vi "Drivetrain Trapezoidal Loop.vi"(9 "Axes":T1) -> (1 "Shift?":bool, 2 "Y Power":dbl)   [LabVIEW 2017]
uses:
  Robot Global Data.vi
  Common Code/Trapezoidal States.ctl
  <vilib>/addons/control/pid/NI_PID_pid.lvlib
  <vilib>/addons/control/pid/pid.llb/PID (DBL).vi
  <vilib>/express/express arith-compare/Formula/XNode/ExpressFormulaBlockNode.xnode
  Common Code/Gamepads/Axes Cluster.ctl
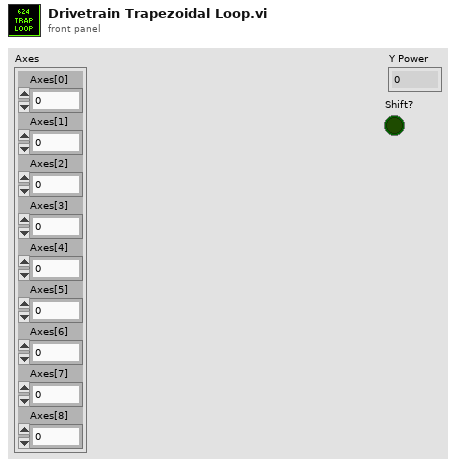
[diagram p1: front panel]
types:
  T1 = typedef "Axes Cluster.ctl" = cluster{"Axes[0]":dbl, "Axes[1]":dbl, "Axes[2]":dbl, "Axes[3]":dbl, "Axes[4]":dbl, "Axes[5]":dbl, "Axes[6]":dbl, "Axes[7]":dbl, "Axes[8]":dbl}
  T2 = typedef "Trapezoidal States.ctl" = enum16{"Feed Forward", "Feed Backwards", "Cruise", "Shift Feed Forward", "Shift Feed Backwards", "Shift Cruise", "Idle"}
  T3 = typedef "Dashboard Control Data.ctl" = cluster{"Drivetrain Settings Cluster":T4, "Intake Presets":T9, "Elevator Settings Cluster":T10, "Drivetrain Encoder Values":T12, "Auton Chooser":T13, "Auton Presets":cluster{"Start Position":dbl}, "Elevator Encoder Values":T14, "Pressure M":dbl, "Pressure B":dbl, "Zero All?":bool, "Enable Vision":bool}
  T4 = typedef "Drivetrain Settings Cluster.ctl" = cluster{"Gyro Steer PID Gains":T5, "Distance Drive PID Gains":T5, "Drive Tolerance":dbl, "Gyro Tolerance":dbl, "Gyro Output":dbl, "Distance Output":dbl, "Y Power Multiplier":dbl, "Turn Power Multiplier":dbl, "Creep Rate":dbl, "Encoder Reset":bool, "DT Mode Modifier":enum16{"None, Default", "Cube", "Square"}, "Left Encoder Tick Constant":dbl, "Right Encoder Tick Constant":dbl, "Shift Speed":dbl, "Zero Gyro":bool, "Y min":dbl, "Y max":dbl, "X min":dbl, "X max":dbl, "Finish Velocity":dbl, "Anti-Tip Settings":T6, "Trapezoidal Settings":T7, "Turning, Don't Shift":dbl}
  T5 = typedef "PID Gains Cluster.ctl" = cluster{"Proportional Gain":dbl, "Integral Time":dbl, "Derivative Time":dbl}
  T6 = typedef "Anti-Tip Settings.ctl" = cluster{"Pitch Tip Constant":dbl, "Wheel Diameter":dbl, "Gearbox Reduction":dbl, "Motor Count":dbl, "Mass of Robot":dbl, "Almost Tip Constant":dbl, "Dist to CG":dbl}
  T7 = typedef "Trapezoidal Settings.ctl" = cluster{"1st Gear Reduction":dbl, "2nd Gear Reduction":dbl, "Maximum RPM":dbl, "1st Gear PVA Gains":T8, "2nd Gear PVA Gains":T8, "Wheel Radius":dbl, "Mass of the Wheel":dbl, "Number of Motors":dbl, "Velocity Tolerance":dbl, "Cruise Time (ms)":dbl, "Efficiency":dbl}
  T8 = typedef "PVA Gains.ctl" = cluster{"Positional Gain":dbl, "Velocity Gain":dbl, "Acceleration Gain":dbl}
  T9 = typedef "Intake Presets.ctl" = cluster{"Idle Angle":dbl, "Mid Angle":dbl, "Low Angle":dbl, "Outtake Power":dbl, "Intake Power":dbl, "Unstuck":dbl, "Angle Tolerance":dbl, "Max Angle":dbl, "Max Current":dbl, "Current Trip Time":dbl, "Reset Encoder?":bool, "Encoder Scale":dbl, "PID gains":cluster{"proportional gain (Kc)":dbl, "integral time (Ti, min)":dbl, "derivative time (Td, min)":dbl}, "output range":cluster{"output high":dbl, "output low":dbl}, "IR Constant Pull Rate":dbl, "Shoot Angle":dbl, "Shoot High":dbl, "Manual Limit":dbl}
  T10 = typedef "Elevator Settings Cluster.ctl" = cluster{"Ground Height":dbl, "Switch Height":dbl, "Scale High Height ":dbl, "Scale Low Height":dbl, "Elevator PID Gains":T11, "Elevator Tolerance":dbl, "Reset Encoders":bool, "Encoder Scale":dbl, "Max Height":dbl, "Mid Height":dbl, "output range":cluster{"output high":dbl, "output low":dbl}, "Upper Slow Down Tolerance":dbl, "Tick Constant":dbl, "Tip Constant":dbl, "Slow Down Multiplier":dbl, "Almost Tip Constant":dbl, "Bottom Trip Offset":dbl, "Lower Slow Down Tolerance":dbl, "Cruise Velocity":dbl, "Max Acceleration":dbl, "Feed Forward":dbl}
  T11 = typedef "PID Gains.ctl" = cluster{"proportional gain (Kc)":dbl, "integral time (Ti, min)":dbl, "derivative time (Td, min)":dbl}
  T12 = typedef "DT Encoder Values.ctl" = cluster{"Left Encoder":cluster{"Distance":dbl, "Speed":dbl, "Tick":dbl}, "Right Encoder":cluster{"Distance":dbl, "Speed":dbl, "Tick":dbl}}
  T13 = typedef "Auton Chooser.ctl" = cluster{"Left":bool, "Center":bool, "Right":bool, "Scale":bool, "Both":bool, "Switch":bool, "Test":bool, "No Script":bool, "Drive PID":bool, "Elevator PID":bool, "Gyro PID":bool, "Drive Forward":bool, "cross front":bool, "Near":bool, "Far":bool, "1 Plus 1":bool, "2 Scale":bool, "2 Switch":bool, "cross behind":bool, "Pick up 2nd cube":bool, "No cross if cross":bool}
  T14 = typedef "Elevator Encoder Values.ctl" = cluster{"Encoder Values":cluster{"Distance":dbl, "Speed":dbl, "Tick":dbl}}
  T15 = typedef "Dashboard Status Data.ctl" = cluster{"Elevator Status Cluster":T16, "Drivetrain Status Cluster":T19, "Intake Status Cluster":T21, "Climb Status Cluster":T24, "Intake PDP Info":T25, "Auton Command Cluster":T26, "Pressure ":dbl, "Auton Field Index":i32, "Auton File Index":i32, "Auton Side Index":i32, "Auton Side":string, "Field Config":string, "Robot Info":T27, "IMU Pitch Zero":dbl, "IMU Roll Zero":dbl, "IMU Yaw Zero":dbl, "Auton Queue Index":i32}
  T16 = typedef "Elevator Status Cluster.ctl" = cluster{"Finished":bool, "Elevator Power":dbl, "Elevator State":T17, "Elevator Mode":T18, "Elevator Height":dbl, "At Bottom?":bool, "At Top?":bool, "Scale high?":bool, "PID Output":dbl, "2nd Gear":bool}
  T17 = typedef "Elevator State.ctl" = enum16{"Idle", "Ground", "Mid", "Scale", "Switch"}
  T18 = typedef "Elevator Mode.ctl" = enum16{"Motion Profile", "Semi Auto", "Manual", "Auto"}
  T19 = typedef "Drivetrain Status Cluster.ctl" = cluster{"Throttle (Y)":dbl, "Steer (X)":dbl, "Drivetrain Mode":T20, "Brake?":bool, "Distance Drive Complete?":bool, "PID Drive Complete?":bool, "Creep Mode?":bool, "Gyro Steer Complete?":bool, "Gyro":dbl, "Heading Target":dbl, "Distance Target":dbl, "2nd Gear":bool, "Drivetrain Encoder Values":T12, "Left Motor Power":dbl, "Right Motor Power":dbl}
  T20 = typedef "Drivetrain Mode.ctl" = enum16{"Manual w/ Autoshift", "Trapezoidal Motion", "Manual", "Gyro Steer", "PID Drive", "Distance Drive", "Autonomous"}
  T21 = typedef "Intake Status Cluster.ctl" = cluster{"Intake Mode":T22, "Intake States":T23, "Intake Current Angle":dbl, "Cube In Posession?":bool, "Intake Wrist Up?":bool, "Right Roller Power":dbl, "Angle Power":dbl, "Left Roller Power":dbl}
  T22 = typedef "Intake Mode.ctl" = enum16{"Auto", "Semi Auto", "Manual"}
  T23 = typedef "Intake States.ctl" = enum16{"Zero", "Override Angle", "Idle", "Drop Mid", "Drop Low", "Outtake", "Intake"}
  T24 = typedef "Climb Status Cluster.ctl" = cluster{"Climb":bool, "Time Remaining":dbl, "Button Pressed":bool}
  T25 = typedef "Intake PDP Info.ctl" = cluster{"Voltage Percent Output":dbl, "Output Voltage":dbl, "Bus Voltage":dbl, "Device ID":dbl, "Output Current":dbl, "Sensor Velocity":dbl, "Sensor Position":dbl, "Pulse Width Position":dbl, "Pulse Width Velocity":dbl, "Temperature":dbl, "Inverted?":bool}
  T26 = typedef "Auton Command Cluster.ctl" = cluster{"commandID":dbl, "headingTarget":dbl, "async":dbl, "elevatorCommand":dbl, "intakeMode":dbl, "maxTime":dbl, "ySpeed":dbl, "zeroGyro":dbl, "intakeCommand":dbl, "distanceTarget":dbl, "xSpeed":dbl, "elevatorMode":dbl, "scaleHigh":dbl, "rollerSpeed":dbl, "intakeAngle":dbl, "manualOpen":dbl, "secondGear":dbl, "elevatorPower":dbl, "waitFor":dbl, "overrideAngle":dbl}
  T27 = typedef "Robot Info.ctl" = cluster{"FMS":bool, "Switch and Scale Sides":string, "Event Name":string, "Alliance":T28, "Position":T29, "Match Number":u16, "Robot Mode":T30, "Match Time(s)":sgl}
  T28 = typedef "WPI_DriverStationAllianceInfo.ctl" = enum16{"Red", "Blue", "Invalid"}
  T29 = typedef "WPI_DriverStationPositionInfo.ctl" = enum16{"1", "2", "3"}
  T30 = typedef "WPI_DriverStationRobotMode2.ctl" = enum16{"Autonomous Disabled", "Autonomous Enabled", "Teleop Disabled", "Teleop Enabled", "Disconnected", "Finish", "Test Disabled", "Test Enabled", "Emergency Stopped"}
  T31 = typedef "Drivetrain Command Cluster.ctl" = cluster{"Y Power":dbl, "Turn Power":dbl, "Drivetrain Mode":T20, "2nd Gear":bool, "Y Min Output":dbl, "Y Max Output":dbl, "X Min Output":dbl, "X Max Output":dbl, "Heading Target":dbl, "Distance Target":dbl, "Brake?":bool, "Zero Gyro":bool, "Trapezoidal States":T2}
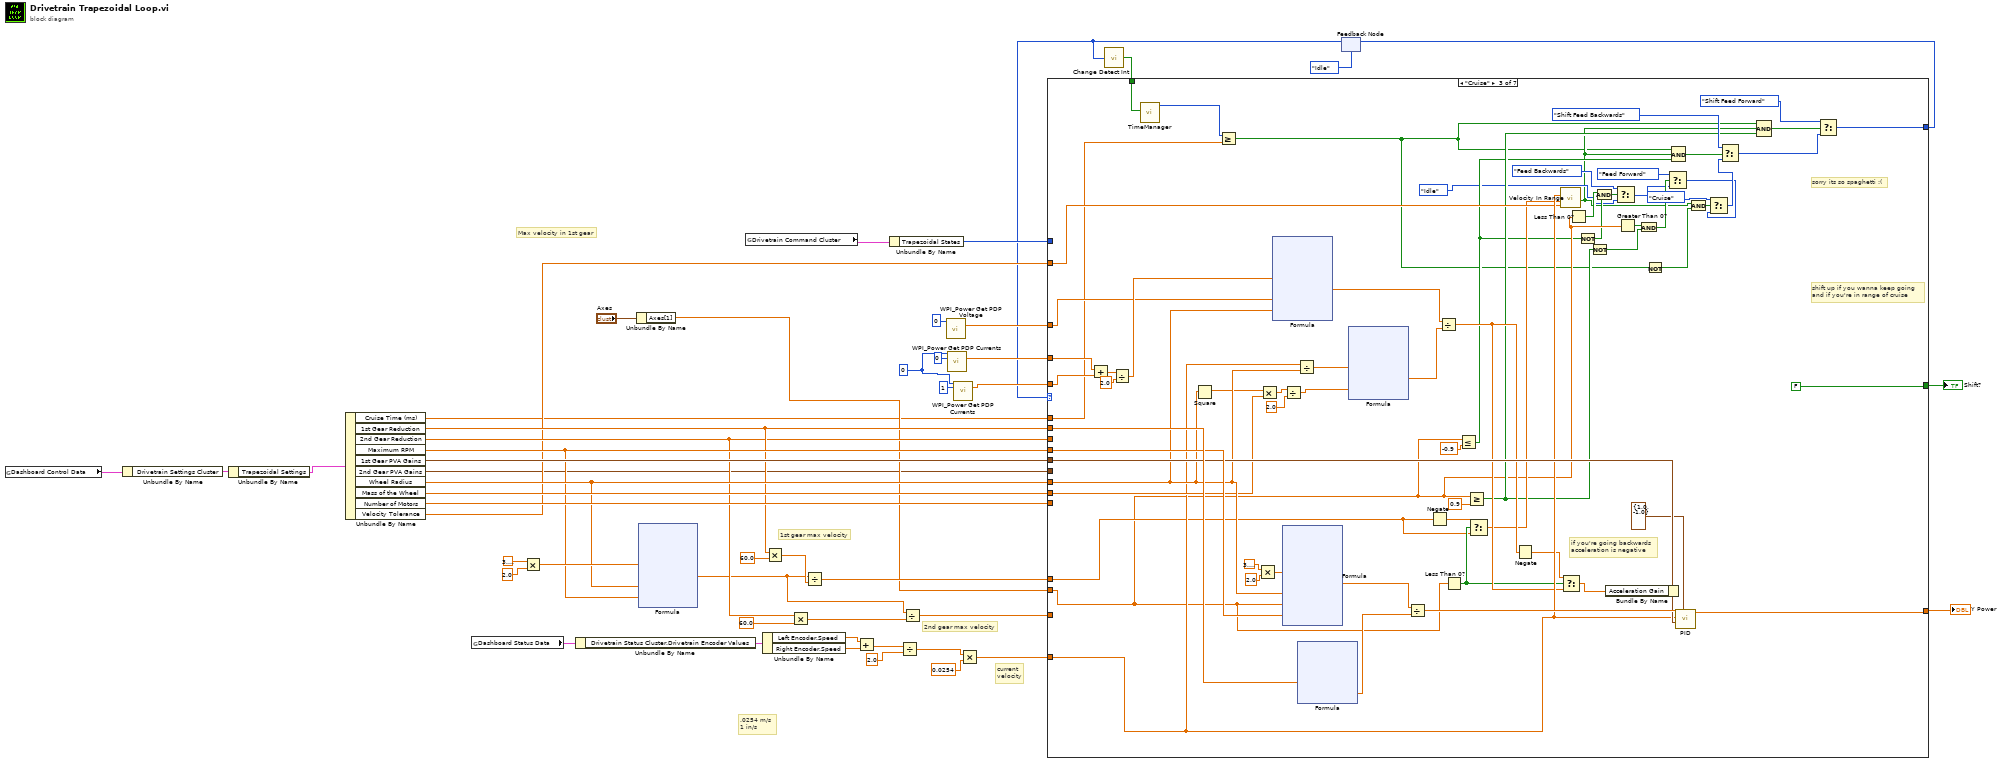
[diagram p0: block diagram]
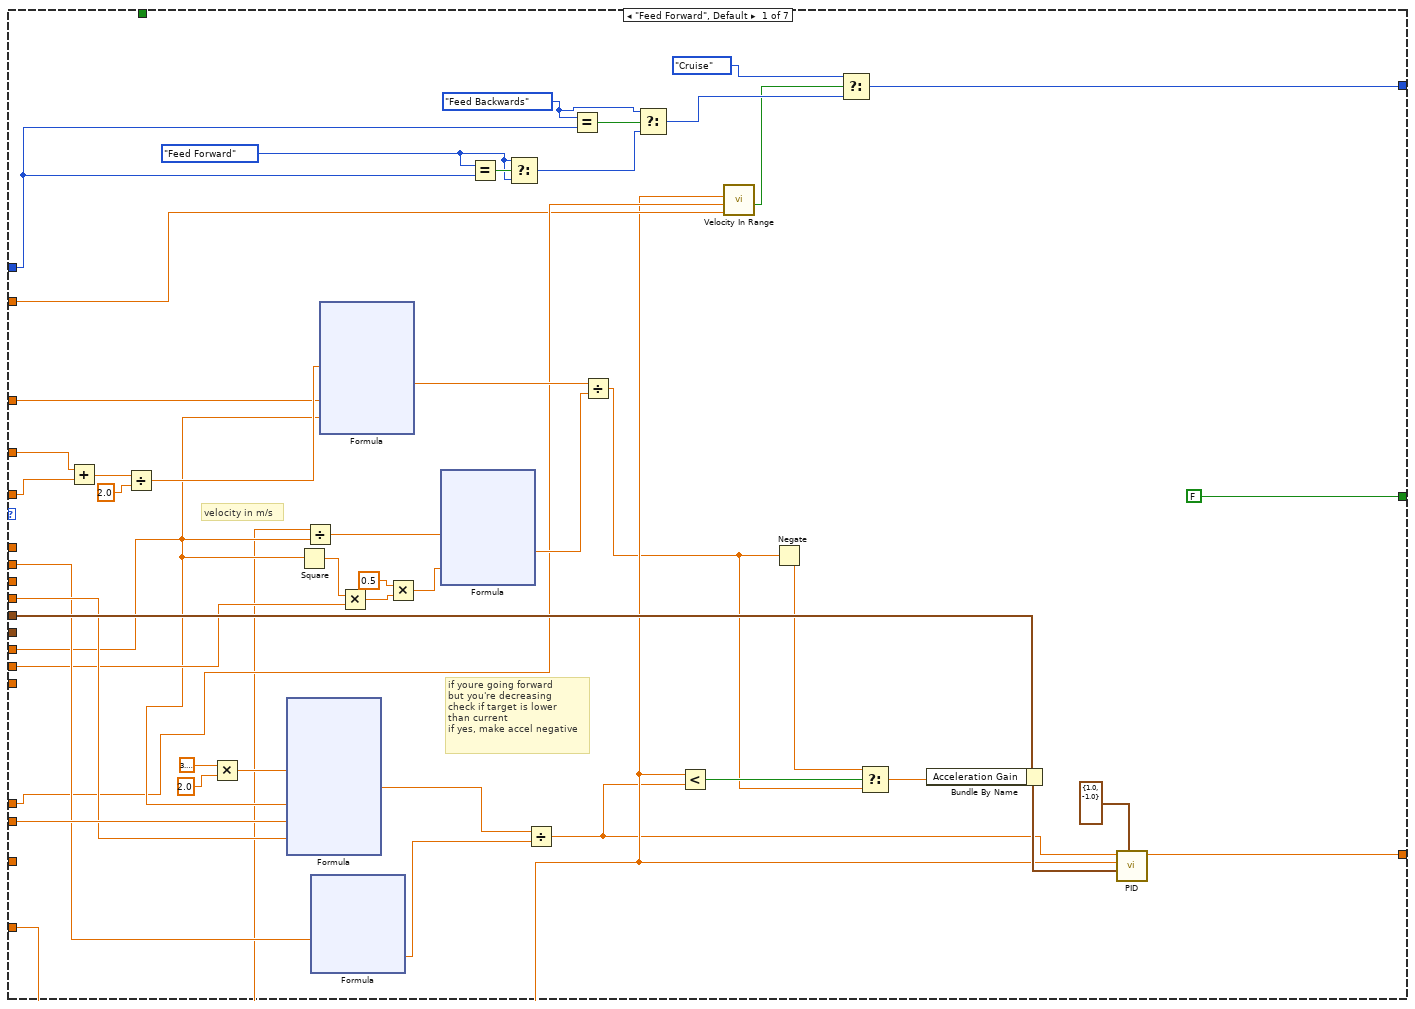
[diagram p2: hidden frame]
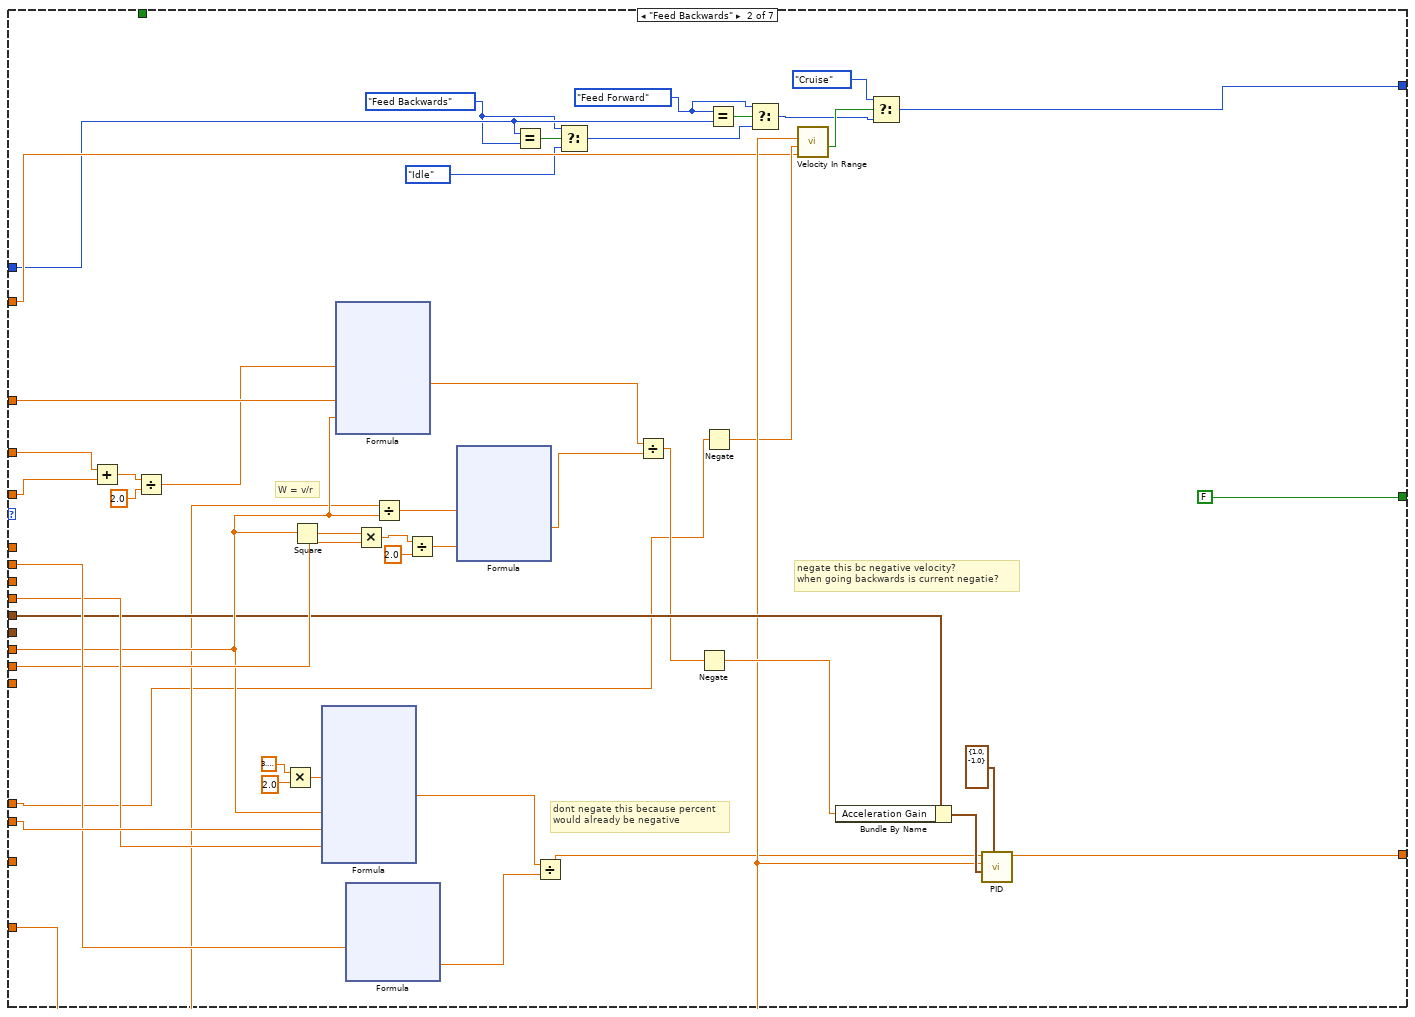
[diagram p3: hidden frame]
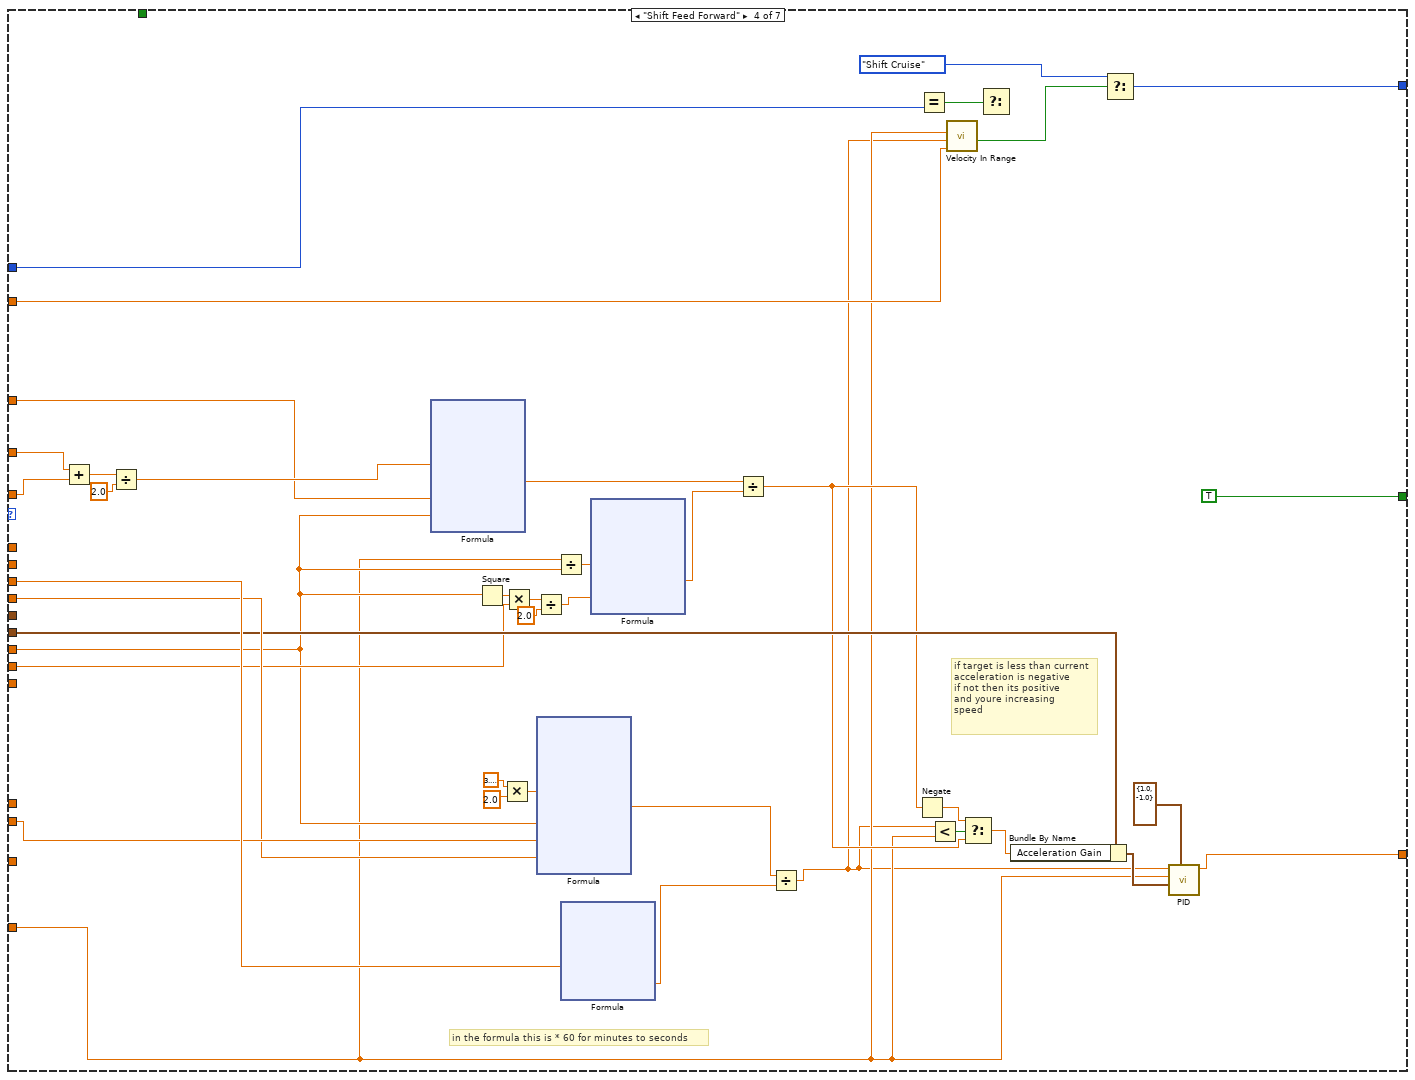
[diagram p4: hidden frame]
diagram:
  w27 = 0
  # "current\nvelocity"
  # "2nd gear max velocity"
  # "1st gear max velocity"
  # "Max velocity in 1st gear"
  # ".0254 m/s \n1 in/s"
  n1 = global read "Robot Global Data.vi" "Dashboard Control Data"() -> (w49:T3)
  n2 = Unbundle By Name(w49) -> ("Drivetrain Settings Cluster"=w48:T4)
  n3 = Unbundle By Name(w48) -> ("Trapezoidal Settings"=w47:T7)
  n4 = Unbundle By Name(w47) -> ("Cruise Time (ms)"=w2:dbl, "1st Gear Reduction"=w19:dbl, "2nd Gear Reduction"=w15:dbl, "Maximum RPM"=w20:dbl, "1st Gear PVA Gains"=w44:T8, "2nd Gear PVA Gains"=w1:T8, "Wheel Radius"=w21:dbl, "Mass of the Wheel"=w43:dbl, "Number of Motors"=w34:dbl, "Velocity Tolerance"=w6:dbl)
  n5 = global read "Robot Global Data.vi" "Dashboard Status Data"() -> (w42:T15)
  n6 = Multiply(x=3.141592653589793, y=2.0) -> (x*y=w23:dbl)
  n7 = Unbundle By Name(w42) -> ("Drivetrain Status Cluster.Drivetrain Encoder Values"=w41:T12)
  n8 = Unbundle By Name("Axes") -> ("Axes[1]"=w8:dbl)
  n9 = xnode "Formula"("2PI"=w23, "Wheel Radius"=w21, "Max RPM"=w20) -> ("Result"=w13:dbl)  [unwired: 1 in, 1 out]
  n10 = global read "Robot Global Data.vi" "Drivetrain Command Cluster"() -> (w46:T31)
  n11 = Unbundle By Name(w41) -> ("Left Encoder.Speed"=w40:dbl, "Right Encoder.Speed"=w39:dbl)
  n12 = Multiply(x=w19, y=60.0) -> (x*y=w17:dbl)
  n13 = Multiply(x=w15, y=60.0) -> (x*y=w12:dbl)
  n14 = Divide(x=w13, y=w17) -> (x/y=w16:dbl)
  n15 = Add(x=w40, y=w39) -> (x+y=w38:dbl)
  n16 = Unbundle By Name(w46) -> ("Trapezoidal States"=w25:T2)
  n17 = Divide(x=w38, y=2.0) -> (x/y=w36:dbl)
  n18 = Divide(x=w13, y=w12) -> (x/y=w11:dbl)
  n19 = call <vilib>:"WPI_Power Get PDP Voltage.vi"("Power Distribution Panel (0)"=u8 0) -> ("voltage (V)"=w31:dbl)  [unwired: 13 in, 1 out]
  n20 = call <vilib>:"WPI_Power Get PDP Currents.vi"("Power Distribution Panel (0)"=w27, "PDP Channel"=0) -> ("current (A)"=w32:dbl)  [unwired: 11 in, 2 out]
  n21 = call <vilib>:"WPI_Power Get PDP Currents.vi"("Power Distribution Panel (0)"=w27, "PDP Channel"=1) -> ("current (A)"=w26:dbl)  [unwired: 11 in, 2 out]
  n22 = Multiply(x=w36, y=0.0254) -> (x*y=w33:dbl)
  n23 = feedback #1(Trapezoidal_States."Idle" ("Trapezoidal States")) -> (w4:T2)
  n24 = call "Change Detect Int.vi"("In"=w4) -> ("Changed?"=w3:bool)
  n25 = case shown="\"Cruise\"" w4 {
    tunnel: w44 -> [w94 w162 w287 _ _ _ _]
    tunnel: w21 -> [w74 w164 w279 w356 _ _ _]
    tunnel: w43 -> [w77 w167 w277 w358 _ _ _]
    tunnel: w20 -> [w89 w179 w295 w375 _ _ _]
    tunnel: w15 -> [_ _ _ w380 _ _ _]
    tunnel: w19 -> [w87 w180 w296 _ _ _ _]
    tunnel: w8 -> [w90 w181 w244 w376 _ _ _]
    tunnel: w34 -> [_ _ _ _ _ _ _]
    tunnel: w33 -> [w55 w155 w271 w345 _ _ _]
    tunnel: w32 -> [w84 w175 w286 w368 _ _ _]
    tunnel: w31 -> [w79 w176 w281 w357 _ _ _]
    tunnel: w26 -> [w83 w174 w285 w367 _ _ _]
    tunnel: w25 -> [w70 w145 _ w342 _ _ _]
    tunnel: w16 -> [w59 w154 w260 _ _ _ _]
    tunnel: w11 -> [_ _ _ _ _ _ _]
    tunnel: [w65 w151 w256 w347 _ _ _] -> w10
    tunnel: [w63 w185 w297 w371 _ _ _] -> w7
    tunnel: w6 -> [w58 w152 w270 w346 _ _ _]
    tunnel: [FALSE FALSE FALSE TRUE _ _ _] -> w5
    tunnel: w3 -> [_ _ w255 _ _ _ _]
    tunnel: w2 -> [_ _ w253 _ _ _ _]
    tunnel: w1 -> [_ _ _ w369 _ _ _]
    frame "Feed Forward", Default {
      w64 = Trapezoidal_States."Feed Forward" ("Trapezoidal States")
      w68 = Trapezoidal_States."Feed Backwards" ("Trapezoidal States")
      # "if youre going forward\nbut you're decreasing\ncheck if target is lower\nthan current \nif yes, make accel negative"
      # "velocity in m/s"
      n26 = Add(x=w84, y=w83) -> (x+y=w82:dbl)
      n27 = Divide(x=w82, y=2.0) -> (x/y=w80:dbl)
      n28 = Multiply(x=3.141592653589793, y=2.0) -> (x*y=w91:dbl)
      n29 = xnode "Formula"("2PI"=w91, "Wheel Radius"=w74, "Percent Output"=w90, "Maximum RPM"=w89) -> ("Result"=w88:dbl)  [unwired: 1 in, 1 out]
      n30 = Square(x=w74) -> (x^2=w62:dbl)
      n31 = Divide(x=w55, y=w74) -> (x/y=w73:dbl)
      n32 = xnode "Formula"("Gear Reduction"=w87) -> ("Result"=w86:dbl)  [unwired: 1 in, 1 out]
      n33 = xnode "Formula"("AvgCurrent"=w80, "Voltage"=w79, "Wheel Radius"=w74) -> ("Result"=w78:dbl)  [unwired: 1 in, 1 out]
      n34 = Multiply(x=w62, y=w77) -> (x*y=w60:dbl)
      n35 = Multiply(x=0.5, y=w60) -> (x*y=w76:dbl)
      n36 = xnode "Formula"("AngularSpeed"=w73, "Inertia"=w76) -> ("Result"=w75:dbl)  [unwired: 1 in, 1 out]
      n37 = Equal?(x=w64, y=w70) -> (x = y?=w69:bool)
      n38 = Select(t=w64, s=w69, f=w64) -> (s? t:f=w66:T2)
      n39 = Divide(x=w88, y=w86) -> (x/y=w54:dbl)
      n40 = Equal?(x=w68, y=w70) -> (x = y?=w71:bool)
      n41 = Divide(x=w78, y=w75) -> (x/y=w50:dbl)
      n42 = Select(t=w68, s=w71, f=w66) -> (s? t:f=w67:T2)
      n43 = Less?(x=w55, y=w54) -> (x < y?=w53:bool)
      n44 = call "Velocity In Range.vi"("Velocity Tolerance"=w58, "Target Velocity"=w59, "Current Velocity"=w55) -> ("In Range?"=w57:bool)  [unwired: 8 in]
      n45 = Negate(x=w50) -> (-x=w52:dbl)
      n46 = Select(t=Trapezoidal_States."Cruise" ("Trapezoidal States"), s=w57, f=w67) -> (s? t:f=w65:T2)
      n47 = Select(t=w52, s=w53, f=w50) -> (s? t:f=w51:dbl)
      n48 = Bundle By Name(cluster=w94, "Acceleration Gain"=w51) -> (w95:T8)
      n49 = call-poly <vilib>:"PID.vi"("output range"=cluster{"output high":dbl, "output low":dbl} {"output high"=1.0, "output low"=-1.0}, "PID gains"=w95, "process variable"=w55, "setpoint"=w54) -> ("output"=w63:dbl)  [unwired: 6 in, 1 out]
    }
    frame "Feed Backwards" {
      w144 = Trapezoidal_States."Feed Backwards" ("Trapezoidal States")
      w148 = Trapezoidal_States."Feed Forward" ("Trapezoidal States")
      # "negate this bc negative velocity?\nwhen going backwards is current negatie?"
      # "dont negate this because percent\nwould already be negative"
      # "W = v/r"
      n50 = Add(x=w175, y=w174) -> (x+y=w173:dbl)
      n51 = Divide(x=w173, y=2.0) -> (x/y=w171:dbl)
      n52 = Multiply(x=3.141592653589793, y=2.0) -> (x*y=w183:dbl)
      n53 = Square(x=w164) -> (x^2=w168:dbl)
      n54 = xnode "Formula"("2PI"=w183, "Wheel Radius"=w164, "Percent Output"=w181, "Maximum RPM"=w179) -> ("Result"=w178:dbl)  [unwired: 1 in, 1 out]
      n55 = xnode "Formula"("AvgCurrent"=w171, "Voltage"=w176, "Wheel Radius"=w164) -> ("Result"=w160:dbl)  [unwired: 1 in, 1 out]
      n56 = xnode "Formula"("Gear Reduction"=w180) -> ("Result"=w177:dbl)  [unwired: 1 in, 1 out]
      n57 = Multiply(x=w168, y=w167) -> (x*y=w166:dbl)
      n58 = Divide(x=w155, y=w164) -> (x/y=w165:dbl)
      n59 = Divide(x=w166, y=2.0) -> (x/y=w170:dbl)
      n60 = xnode "Formula"("AngularSpeed"=w165, "Inertia"=w170) -> ("Result"=w159:dbl)  [unwired: 1 in, 1 out]
      n61 = Equal?(x=w145, y=w144) -> (x = y?=w146:bool)
      n62 = Divide(x=w178, y=w177) -> (x/y=w150:dbl)
      n63 = Select(t=w144, s=w146, f=Trapezoidal_States."Idle" ("Trapezoidal States")) -> (s? t:f=w143:T2)
      n64 = Divide(x=w160, y=w159) -> (x/y=w158:dbl)
      n65 = Negate(x=w158) -> (-x=w161:dbl)
      n66 = Negate(x=w154) -> (-x=w153:dbl)
      n67 = Equal?(x=w148, y=w145) -> (x = y?=w149:bool)
      n68 = Select(t=w148, s=w149, f=w143) -> (s? t:f=w147:T2)
      n69 = call "Velocity In Range.vi"("Velocity Tolerance"=w152, "Target Velocity"=w153, "Current Velocity"=w155) -> ("In Range?"=w156:bool)  [unwired: 8 in]
      n70 = Bundle By Name(cluster=w162, "Acceleration Gain"=w161) -> (w163:T8)
      n71 = Select(t=Trapezoidal_States."Cruise" ("Trapezoidal States"), s=w156, f=w147) -> (s? t:f=w151:T2)
      n72 = call-poly <vilib>:"PID.vi"("output range"=cluster{"output high":dbl, "output low":dbl} {"output high"=1.0, "output low"=-1.0}, "PID gains"=w163, "process variable"=w155, "setpoint"=w150) -> ("output"=w185:dbl)  [unwired: 6 in, 1 out]
    }
    frame "Cruise" {
      # "sorry its so spaghetti :("
      # "if you're going backwards\nacceleration is negative"
      # "shift up if you wanna keep going \nand if you're in range of cruise"
      n73 = Add(x=w286, y=w285) -> (x+y=w284:dbl)
      n74 = Divide(x=w284, y=2.0) -> (x/y=w282:dbl)
      n75 = call "TimeManager.vi"("Reset?"=w255) -> ("Time Since Reset"=w254:u32)  [unwired: 9 in, 1 out]
      n76 = Square(x=w279) -> (x^2=w278:dbl)
      n77 = Greater Or Equal?(x=w254, y=w253) -> (x >= y?=w234:bool)
      n78 = Multiply(x=3.141592653589793, y=2.0) -> (x*y=w294:dbl)
      n79 = Multiply(x=w278, y=w277) -> (x*y=w276:dbl)
      n80 = xnode "Formula"("AvgCurrent"=w282, "Voltage"=w281, "Wheel Radius"=w279) -> ("Result"=w273:dbl)  [unwired: 1 in, 1 out]
      n81 = xnode "Formula"("2PI"=w294, "Wheel Radius"=w279, "Percent Output"=w244, "Maximum RPM"=w295) -> ("Result"=w291:dbl)  [unwired: 1 in, 1 out]
      n82 = Divide(x=w276, y=2.0) -> (x/y=w274:dbl)
      n83 = Divide(x=w271, y=w279) -> (x/y=w280:dbl)
      n84 = xnode "Formula"("Gear Reduction"=w296) -> ("Result"=w290:dbl)  [unwired: 1 in, 1 out]
      n85 = xnode "Formula"("AngularSpeed"=w280, "Inertia"=w274) -> ("Result"=w272:dbl)  [unwired: 1 in, 1 out]
      n86 = Divide(x=w291, y=w290) -> (x/y=w289:dbl)
      n87 = Negate(x=w260) -> (-x=w261:dbl)
      n88 = Divide(x=w273, y=w272) -> (x/y=w266:dbl)
      n89 = Less Than 0?(x=w244) -> (x < 0?=w262:bool)
      n90 = Less Or Equal?(x=w244, y=-0.9) -> (x <= y?=w242:bool)
      n91 = Greater Or Equal?(x=w244, y=0.9) -> (x >= y?=w249:bool)
      n92 = Select(t=w261, s=w262, f=w260) -> (s? t:f=w259:dbl)
      n93 = Negate(x=w266) -> (-x=w267:dbl)
      n94 = call "Velocity In Range.vi"("Velocity Tolerance"=w270, "Target Velocity"=w259, "Current Velocity"=w271) -> ("In Range?"=w235:bool)  [unwired: 8 in]
      n95 = Select(t=w267, s=w262, f=w266) -> (s? t:f=w265:dbl)
      n96 = Less Than 0?(x=w244) -> (x < 0?=w243:bool)
      n97 = Not(x=w242) -> (.not. x?=w241:bool)
      n98 = Not(x=w249) -> (.not. x?=w248:bool)
      n99 = And(x=w243, y=w241) -> (x .and. y?=w245:bool)
      n100 = Bundle By Name(cluster=w287, "Acceleration Gain"=w265) -> (w288:T8)
      n101 = Select(t=Trapezoidal_States."Feed Backwards" ("Trapezoidal States"), s=w245, f=Trapezoidal_States."Idle" ("Trapezoidal States")) -> (s? t:f=w239:T2)
      n102 = Greater Than 0?(x=w244) -> (x > 0?=w250:bool)
      n103 = And(x=w250, y=w248) -> (x .and. y?=w247:bool)
      n104 = Not(x=w234) -> (.not. x?=w233:bool)
      n105 = Select(t=Trapezoidal_States."Feed Forward" ("Trapezoidal States"), s=w247, f=w239) -> (s? t:f=w230:T2)
      n106 = Compound Arithmetic op=AND(w234, w235, w242) -> (w251:bool)
      n107 = call-poly <vilib>:"PID.vi"("output range"=cluster{"output high":dbl, "output low":dbl} {"output high"=1.0, "output low"=-1.0}, "PID gains"=w288, "process variable"=w271, "setpoint"=w289) -> ("output"=w297:dbl)  [unwired: 6 in, 1 out]
      n108 = And(x=w235, y=w233) -> (x .and. y?=w236:bool)
      n109 = Select(t=Trapezoidal_States."Cruise" ("Trapezoidal States"), s=w236, f=w230) -> (s? t:f=w231:T2)
      n110 = Select(t=Trapezoidal_States."Shift Feed Backwards" ("Trapezoidal States"), s=w251, f=w231) -> (s? t:f=w257:T2)
      n111 = Compound Arithmetic op=AND(w234, w235, w249) -> (w252:bool)
      n112 = Select(t=Trapezoidal_States."Shift Feed Forward" ("Trapezoidal States"), s=w252, f=w257) -> (s? t:f=w256:T2)
    }
    frame "Shift Feed Forward" {
      # "in the formula this is * 60 for minutes to seconds"
      # "if target is less than current\nacceleration is negative \nif not then its positive \nand youre increasing\nspeed"
      n113 = Add(x=w368, y=w367) -> (x+y=w366:dbl)
      n114 = Divide(x=w366, y=2.0) -> (x/y=w364:dbl)
      n115 = xnode "Formula"("AvgCurrent"=w364, "Voltage"=w357, "Wheel Radius"=w356) -> ("Result"=w355:dbl)  [unwired: 1 in, 1 out]
      n116 = Square(x=w356) -> (x^2=w359:dbl)
      n117 = Multiply(x=3.141592653589793, y=2.0) -> (x*y=w379:dbl)
      n118 = Multiply(x=w359, y=w358) -> (x*y=w362:dbl)
      n119 = Divide(x=w362, y=2.0) -> (x/y=w361:dbl)
      n120 = xnode "Formula"("2PI"=w379, "Wheel Radius"=w356, "Percent Output"=w376, "Maximum RPM"=w375) -> ("Result"=w374:dbl)  [unwired: 1 in, 1 out]
      n121 = Divide(x=w345, y=w356) -> (x/y=w363:dbl)
      n122 = xnode "Formula"("Gear Reduction"=w380) -> ("Result"=w373:dbl)  [unwired: 1 in, 1 out]
      n123 = xnode "Formula"("AngularSpeed"=w363, "Inertia"=w361) -> ("Result"=w354:dbl)  [unwired: 1 in, 1 out]
      n124 = Divide(x=w355, y=w354) -> (x/y=w351:dbl)
      n125 = Divide(x=w374, y=w373) -> (x/y=w344:dbl)
      n126 = Negate(x=w351) -> (-x=w352:dbl)
      n127 = Equal?(y=w342) -> (x = y?=w343:bool)  [unwired: 1 in]
      n128 = Less?(x=w344, y=w345) -> (x < y?=w353:bool)
      n129 = call "Velocity In Range.vi"("Velocity Tolerance"=w346, "Target Velocity"=w344, "Current Velocity"=w345) -> ("In Range?"=w349:bool)  [unwired: 8 in]
      n130 = Select(t=w352, s=w353, f=w351) -> (s? t:f=w350:dbl)
      n131 = Select(s=w343) -> ()  [unwired: 2 in, 1 out]
      n132 = Bundle By Name(cluster=w369, "Acceleration Gain"=w350) -> (w370:T8)
      n133 = Select(t=Trapezoidal_States."Shift Cruise" ("Trapezoidal States"), s=w349) -> (s? t:f=w347:T2)  [unwired: 1 in]
      n134 = call-poly <vilib>:"PID.vi"("output range"=cluster{"output high":dbl, "output low":dbl} {"output high"=1.0, "output low"=-1.0}, "PID gains"=w370, "process variable"=w345, "setpoint"=w344) -> ("output"=w371:dbl)  [unwired: 6 in, 1 out]
    }
    frame "Shift Feed Backwards" {
    }
    frame "Shift Cruise" {
    }
    frame "Idle" {
    }
  }
  "Y Power" <- w7
  "Shift?" <- w5
  n135 = feedback-in #1(w10) -> ()
